vi "zc_ys.vi"(0 "action":string, 1 "LabVIEW Web Service Request":refnum<class "Web Request.lvclass"> caption="LabVIEW Web服务请求", 3 "sp_yijian":string, 4 "key":string, 5 "id":string, 7 "zc_luodi_num":string, 8 "sp_shuoming":string, 9 "didian":string, 13 "shuoming":string, 14 "lc_num":string) -> (15 "error":errorcluster)   [LabVIEW 2017]
uses:
  <vilib>/wsapi/Web Request.lvclass
panel:
  in  "error 4":errorcluster={"status"=TRUE, "code"=254, "source"="您无权申请该流程！"} caption="error"
  in  "error 3":errorcluster={"status"=TRUE, "code"=255, "source"="当前资产不是“待验收”状态！"} caption="error"
  out "postdata":string caption="post数据"
  out "error out":errorcluster caption="错误输出"
  # "Web服务请求输入接线端用于调用“Web服务”选板的VI。除非不需要访问该选板，否则不要在连线板上删除这个输入接线端。"
  # "添加至连线板的每一个其他输入控件，在URL中对应于一个输入。如需在接线端模式输出（默认设置）下包含显示控件，则该显示控件必须与连线板相连。"
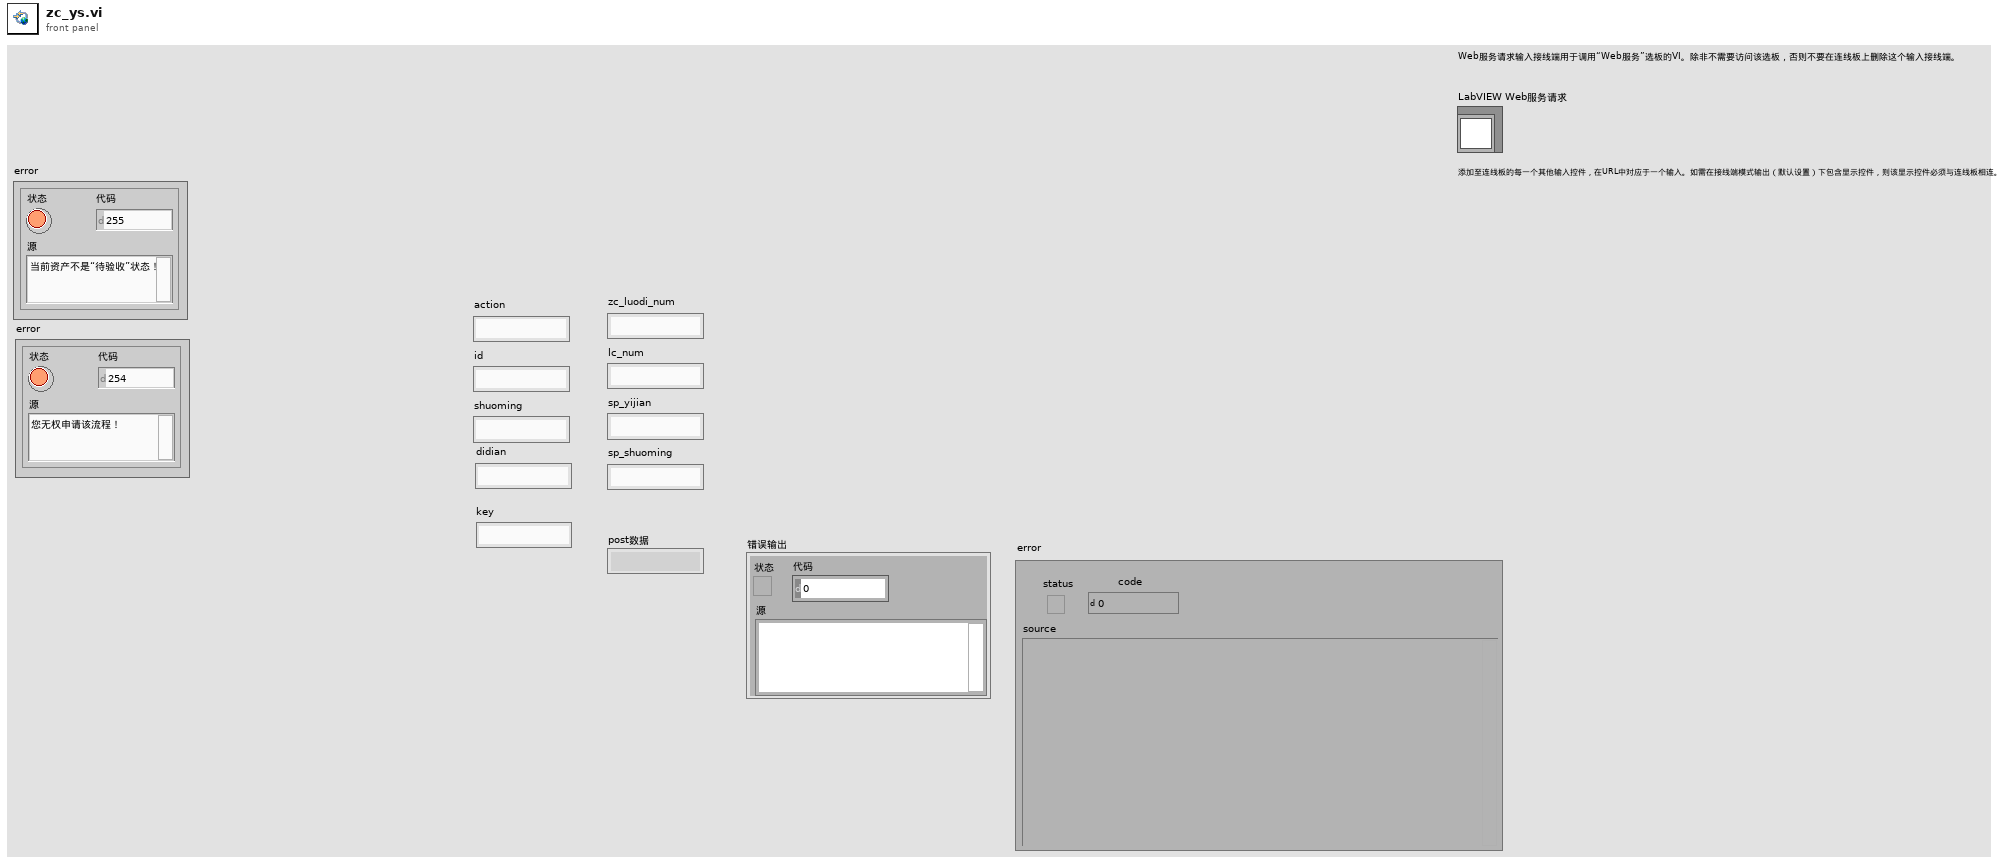
[diagram p1: front panel]
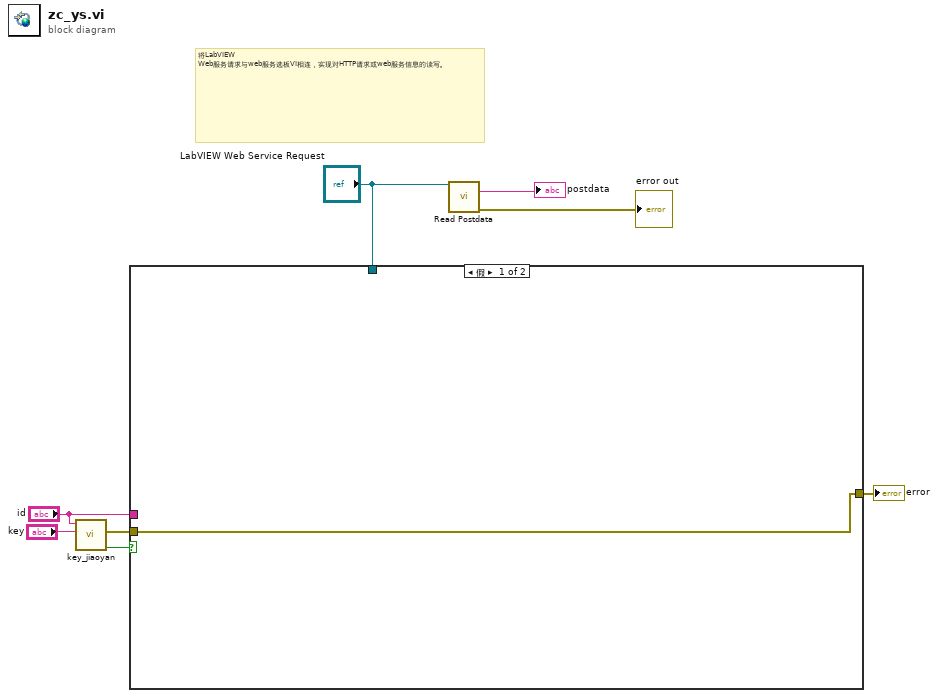
[diagram p0: block diagram]
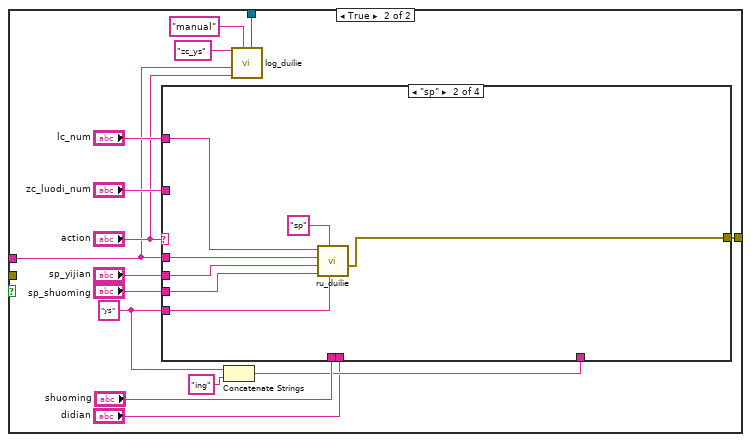
[diagram p2: hidden frame]
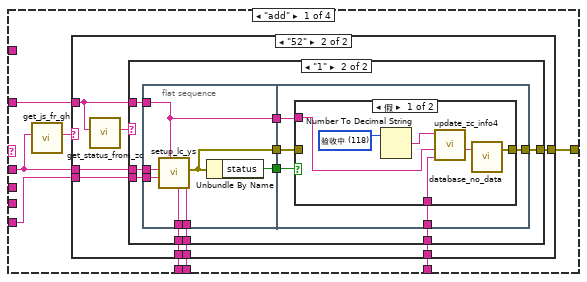
[diagram p3: hidden frame]
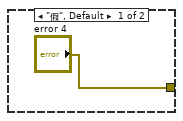
[diagram p4: hidden frame]
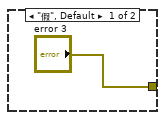
[diagram p5: hidden frame]
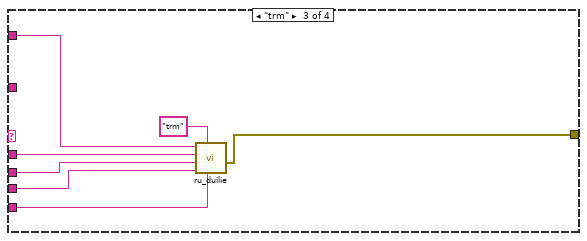
[diagram p7: hidden frame]
diagram:
  # "将LabVIEW Web服务请求与web服务选板VI相连，实现对HTTP请求或web服务信息的读写。"
  n1 = call "key_jiaoyan.vi"("key_client"="key", "gonghao"="id") -> ("jy"=w2:bool, "error"=w1:errorcluster)  [unwired: 8 in]
  n2 = case shown="假" w2 {
    tunnel: [w9 w19] -> w7
    tunnel: "LabVIEW Web Service Request" -> [_ w12]
    tunnel: "id" -> [_ w10]
    tunnel: w1 -> [w9 _]
    frame False {
    }
    frame True {
      w17 = "ys" ("yw")
      n3 = Concatenate Strings(w17, "ing" ("字符串")) -> (w16:string)
      n4 = case shown="\"sp\"" "action" {
        tunnel: w10 -> [w26 w77 w84 _]
        tunnel: "zc_luodi_num" -> [w27 _ _ _]
        tunnel: "sp_yijian" -> [_ w75 w82 _]
        tunnel: "sp_shuoming" -> [_ w74 w81 _]
        tunnel: "shuoming" -> [w32 _ _ _]
        tunnel: w17 -> [w31 w73 w80 _]
        tunnel: "lc_num" -> [_ w76 w83 _]
        tunnel: [w30 w72 w79 _] -> w19
        tunnel: w16 -> [w29 _ _ _]
        tunnel: "didian" -> [w28 _ _ _]
        frame "add" {
          n5 = call "get_js_fr_gh.vi"("gonghao"=w26) -> ("juese"=w25:string)  [unwired: 9 in, 1 out]
          n6 = case shown="\"52\"" w25 {
            tunnel: w32 -> [_ w41]
            tunnel: w31 -> [_ w40]
            tunnel: ["error 4" w39] -> w30
            tunnel: w29 -> [_ w38]
            tunnel: w28 -> [_ w37]
            tunnel: w27 -> [_ w36]
            tunnel: w26 -> [_ w34]
            frame "假", Default {
            }
            frame "52" {
              n7 = call "get_status_from_zc.vi"("zc_luodi_num"=w36) -> ("status"=w35:string)  [unwired: 9 in, 1 out]
              n8 = case shown="\"1\"" w35 {
                tunnel: w41 -> [_ w51]
                tunnel: w34 -> [_ w50]
                tunnel: w40 -> [_ w49]
                tunnel: ["error 3" w48] -> w39
                tunnel: w38 -> [_ w47]
                tunnel: w37 -> [_ w46]
                tunnel: w36 -> [_ w45]
                frame "假", Default {
                }
                frame "1" {
                  n9 = flat-sequence {
                    tunnel: w51 -> [w56]
                    tunnel: w45 -> [w59]
                    tunnel: w50 -> [w58]
                    tunnel: w49 -> [w55]
                    tunnel: [w59] -> w52
                    tunnel: w46 -> [w57]
                    tunnel: [w54] -> w44
                    tunnel: [w53] -> w43
                    tunnel: w52 -> [w63]
                    tunnel: [w64] -> w48
                    tunnel: w47 -> [w62]
                    tunnel: w44 -> [w61]
                    tunnel: w43 -> [w60]
                    frame #0 {
                      n10 = call "setup_lc_ys.vi"("didian"=w57, "shuoming"=w56, "zc_luodi_num"=w59, "yw"=w55, "id"=w58) -> ("error"=w53:errorcluster)  [unwired: 6 in]
                      n11 = Unbundle By Name(w53) -> ("status"=w54:bool)
                    }
                    frame #1 {
                      n12 = case shown="假" w61 {
                        tunnel: [w68 w71] -> w64
                        tunnel: w63 -> [w65 _]
                        tunnel: w62 -> [w67 _]
                        tunnel: w60 -> [_ w71]
                        frame False {
                          w70 = u8 118 items=["待验收"=1, "无需验收"=2, "验收不合格"=3, "待入库"=4, "入库"=5, "领用"=6, "借用"=7, "托管"=8, "接管"=9, "退出"=10, "出库在用"=11, "盘亏"=12, "出售"=13, "报废"=14, "验收中"=118, "入库中"=119, "领用中"=120, "退库中"=121, "借用中"=122, "归还中"=123, "转移中"=124, "调拨中"=125, "借调中"=126, "托管中"=127, "终止托管中"=128, "退出中"=129, "处置中"=130] ("状态选择器")
                          n13 = Number To Decimal String(number=w70) -> (decimal integer string=w66:string)  [unwired: 1 in]
                          n14 = call "update_zc_info4.vi"("ywxinxi"=w67, "number"=w65, "status"=w66) -> ("data_str"=w69:string)  [unwired: 8 in]
                          n15 = call "database_no_data.vi"("input"=w69) -> ("error"=w68:errorcluster)  [unwired: 2 in]
                        }
                        frame True {
                        }
                      }
                    }
                  }
                }
              }
            }
          }
        }
        frame "sp" {
          n16 = call "ru_duilie.vi"("yw"=w73, "name"="sp" ("元素"), "sp_shuoming"=w74, "sp_yijian"=w75, "id"=w77, "lc_num"=w76) -> ("error"=w72:errorcluster)  [unwired: 5 in]
        }
        frame "trm" {
          n17 = call "ru_duilie.vi"("yw"=w80, "name"="trm" ("元素"), "sp_shuoming"=w81, "sp_yijian"=w82, "id"=w84, "lc_num"=w83) -> ("error"=w79:errorcluster)  [unwired: 5 in]
        }
        frame Default {
        }
      }
      n18 = call "log_duilie.vi"("LabVIEW Web Service Request"=w12, "type"="manual", "action"="action", "user"=w10, "yw"="zc_ys") -> ()  [unwired: 7 in]
    }
  }
  "error" <- w7
  n19 = call <vilib>:"Read Postdata.vi"("LabVIEW Web Service Request"="LabVIEW Web Service Request") -> ("postdata"=→"postdata":string, "error out"=→"error out":errorcluster)  [unwired: 12 in, 1 out]
